vi "Bundle.vi"(8 "error in":errorcluster, 10 "Instrument Alias Array":T1[](array[typedef]), 11 "Instrument Alias Data in":refnum<class "Instrument Alias Data.lvclass">) -> (0 "error out":errorcluster, 3 "Instrument Alias Data out":refnum<class "Instrument Alias Data.lvclass">)   [LabVIEW 2020, in "Instrument Handler.lvlib" / "Instrument Alias Data.lvclass"]
doc: "Populate the Instrument Alias Data."
uses:
  Instrument Alias Data.lvclass
  Controls/Ctl_DriverAliasElement.ctl
  Instrument Alias Data.lvclass/Instrument Alias Data.ctl
  Instrument Handler.lvlib
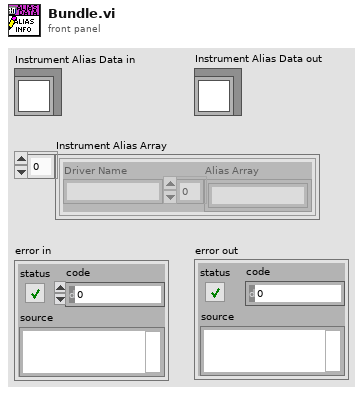
[diagram p1: front panel]
types:
  T1 = typedef "Instrument Handler.lvlib/Ctl_DriverAliasElement.ctl" = cluster{"Driver Name":string, "Alias Array":string[]}
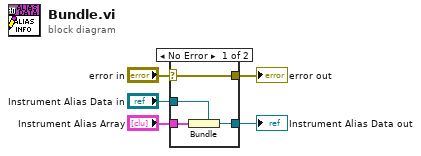
[diagram p0: block diagram]
diagram:
  n1 = case shown="No Error" "error in" {
    selector: "error in" -> [w6 w10]
    tunnel: [w9 w11] -> w5
    tunnel: "Instrument Alias Data in" -> [w8 w11]
    tunnel: "Instrument Alias Array" -> [w7 _]
    tunnel: [w6 w10] -> w1
    frame No Error {
      n2 = Bundle(cluster=w8, w7) -> (w9:refnum<class "Instrument Alias Data.lvclass">)
    }
    frame Error {
    }
  }
  "Instrument Alias Data out" <- w5
  "error out" <- w1
